vi ".vi"(0 "Array":dbl[](array[numeric]), 8 "file path (dialog if empty)":path) -> (7 "Right":cluster{"Y":dbl[], "Y":dbl[]}[](graph), 9 "Right 2":cluster{"Y":dbl[], "Y":dbl[]}[](graph), 10 "3D Graph":refnum<class "Base Datatype.lvclass">[](xcontrol), 11 "origem x":dbl, 12 "Ultimo":dbl[](array[numeric]), 13 "Roots XZ":cdb[](array[numeric]), 14 "Primeiro":dbl[](array[numeric]), 15 "origem y":dbl, 16 "Areas dos triangulos":dbl[](array[numeric]), 17 "Roots YZ":cdb[](array[numeric]), 18 "Top":cluster{"Y":dbl[], "Y":dbl[]}[](graph), 19 "Roots":cdb[](array[numeric]), 20 "chegada":dbl[](array[numeric]), 21 "Top 2":cluster{"Y":dbl[], "Y":dbl[]}[](graph), 22 "partida":dbl[](array[numeric]), 23 "Front":cluster{"Y":dbl[], "Y":dbl[]}[](graph), 24 "3D Graph 2":refnum<class "Base Datatype.lvclass">[](xcontrol), 25 "Front 2":cluster{"Y":dbl[], "Y":dbl[]}[](graph), 26 "origem z":dbl)   [LabVIEW 2019]
uses:
  <vilib>/Native 3D Graph/xcontrol/3DPC_SurfacePlot.xctl
  <vilib>/Analysis/NI_AALPro.lvlib
  <vilib>/Analysis/NI_AAL_Geometry.lvlib
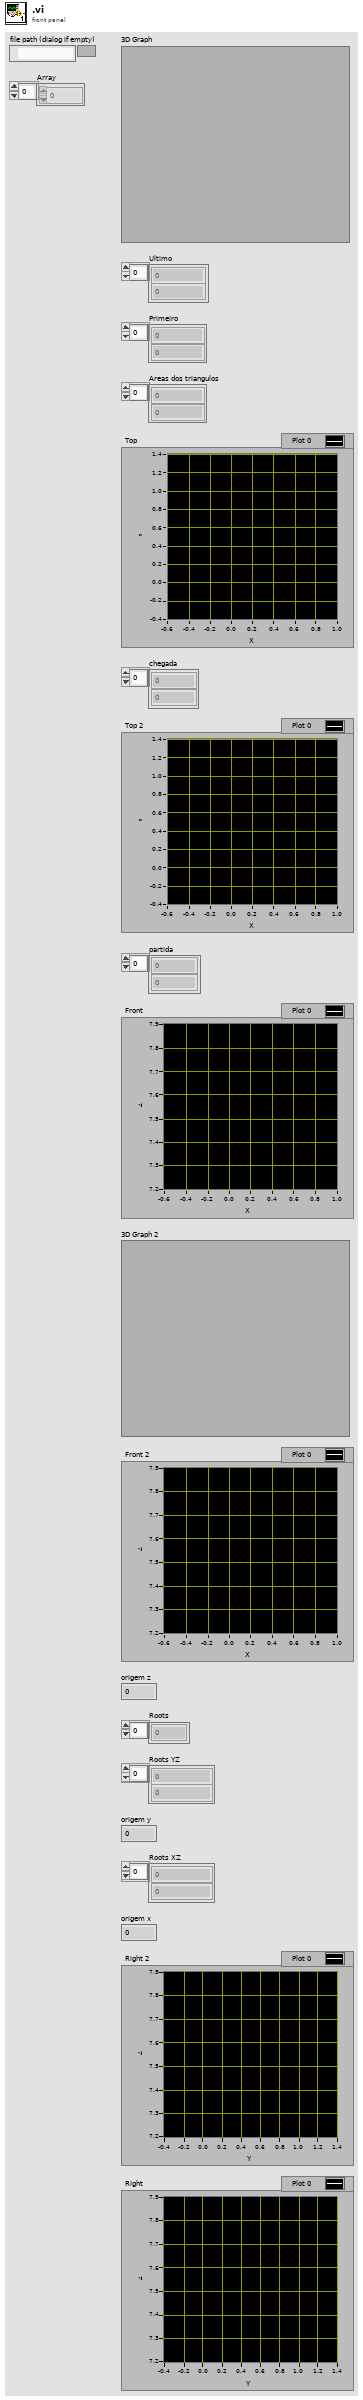
[diagram p1: front panel]
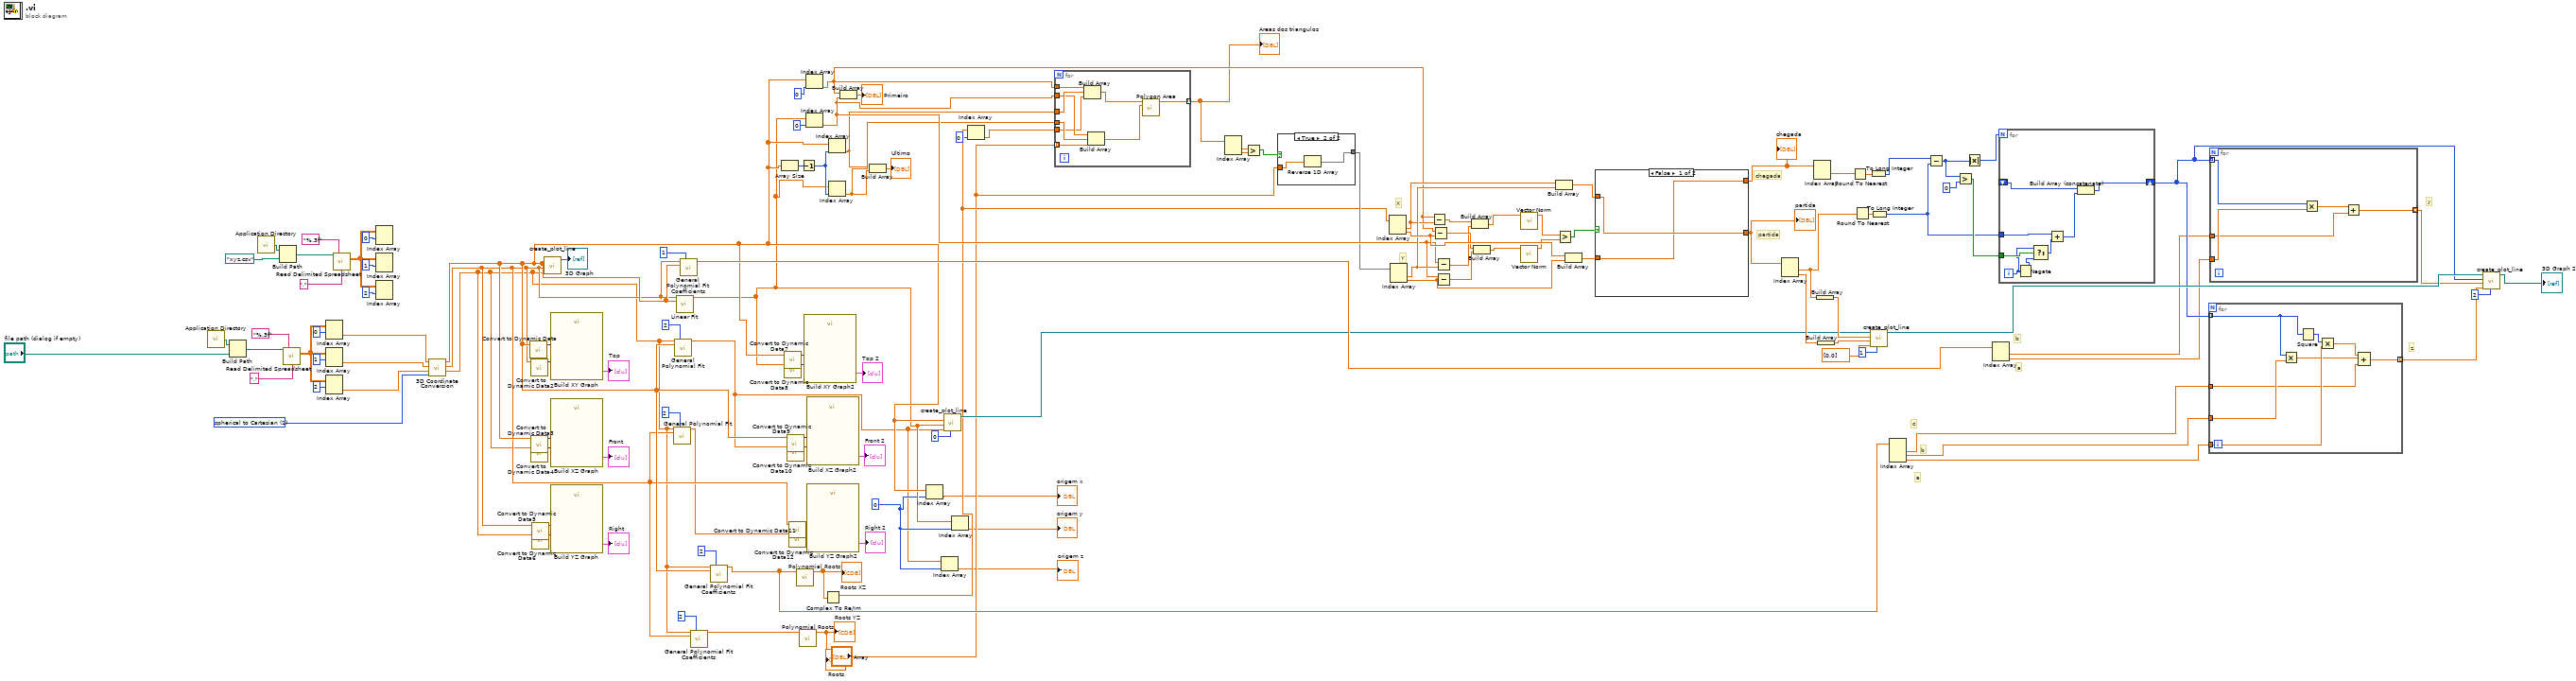
[diagram p0: block diagram]
diagram:
  w53 = 0
  w35 = u16 1 items=["Cartesian to spherical", "spherical to Cartesian", "Cartesian to cylindrical", "cylindrical to Cartesian", "spherical to cylindrical", "cylindrical to spherical"] ("conversion type")
  # "y"
  # "z"
  # "b"
  # "a"
  # "c"
  # "b"
  # "a"
  # "partida"
  # "chegada"
  # "Y"
  # "X"
  n1 = call <vilib>:"Application Directory.vi"() -> ("Application Directory"=w38:path)
  n2 = Build Path(base path=w38, name or relative path="file path (dialog if empty)") -> (appended path=w37:path)
  n3 = call <vilib>:"Application Directory.vi"() -> ("Application Directory"=w3:path)
  n4 = Build Path(base path=w3, name or relative path=path "xyz.csv" ("file path (dialog if empty)")) -> (appended path=w2:path)
  n5 = call-poly <vilib>:"Read Delimited Spreadsheet.vi"("file path (dialog if empty)"=w37, "format (%.3f)"="%.3f", "delimiter (\\t)"="," ("delimiter (\\t)")) -> ("all rows"=w44:dbl[][])  [unwired: 7 in, 5 out]
  n6 = Index Array(array=w44, index (row)=0) -> (element=w48:dbl[])  [unwired: 1 in]
  n7 = Index Array(array=w44, index (row)=1) -> (element=w47:dbl[])  [unwired: 1 in]
  n8 = Index Array(array=w44, index (row)=2) -> (element=w46:dbl[])  [unwired: 1 in]
  n9 = call-poly <vilib>:"Read Delimited Spreadsheet.vi"("file path (dialog if empty)"=w2, "format (%.3f)"="%.3f", "delimiter (\\t)"="," ("delimiter (\\t)")) -> ("all rows"=w10:dbl[][])  [unwired: 7 in, 5 out]
  n10 = Index Array(array=w10, index (row)=0) -> ()  [unwired: 1 in, 1 out]
  n11 = Index Array(array=w10, index (row)=1) -> ()  [unwired: 1 in, 1 out]
  n12 = Index Array(array=w10, index (row)=2) -> ()  [unwired: 1 in, 1 out]
  n13 = call-poly <vilib>:"3D Coordinate Conversion.vi"("conversion type"=w35, "Axis 3"=w46, "Axis 2"=w47, "Axis 1"=w48) -> ("Axis 3 Out"=w45:dbl[], "Axis 2 Out"=w112:dbl[], "Axis 1 Out"=w113:dbl[])  [unwired: 4 in, 1 out]
  n14 = call "Convert to Dynamic Data"("Array"=w113) -> ("Dynamic Data Type"=w12:dynamicdata)  [unwired: 3 in]
  n15 = call "Convert to Dynamic Data2"("Array"=w112) -> ("Dynamic Data Type"=w13:dynamicdata)  [unwired: 3 in]
  n16 = call "Convert to Dynamic Data3"("Array"=w113) -> ("Dynamic Data Type"=w16:dynamicdata)  [unwired: 3 in]
  n17 = call "Convert to Dynamic Data4"("Array"=w45) -> ("Dynamic Data Type"=w17:dynamicdata)  [unwired: 3 in]
  n18 = call "Convert to Dynamic Data5"("Array"=w112) -> ("Dynamic Data Type"=w18:dynamicdata)  [unwired: 3 in]
  n19 = call "Convert to Dynamic Data6"("Array"=w45) -> ("Dynamic Data Type"=w19:dynamicdata)  [unwired: 3 in]
  n20 = call <vilib>:"create_plot_line.vi"("z vector"=w45, "y vector"=w112, "x vector"=w113) -> ("plots out"=→"3D Graph":refnum<class "Base Datatype.lvclass">[])  [unwired: 2 in, 6 out]
  n21 = call "Build XY Graph"("Y Input"=w13, "X Input"=w12) -> ("XY Graph"=→"Top":cluster{"X":dbl[], "Y":dbl[]}[])  [unwired: 8 in, 1 out]
  n22 = call "Build XZ Graph"("Y Input"=w17, "X Input"=w16) -> ("XY Graph"=→"Front":cluster{"X":dbl[], "Y":dbl[]}[])  [unwired: 8 in, 1 out]
  n23 = call "Build YZ Graph"("Y Input"=w19, "X Input"=w18) -> ("XY Graph"=→"Right":cluster{"X":dbl[], "Y":dbl[]}[])  [unwired: 8 in, 1 out]
  n24 = call <vilib>:"General Polynomial Fit.vi"("Y"=w45, "polynomial order"=2, "X"=w112) -> ("Best Polynomial Fit"=w31:dbl[])  [unwired: 9 in, 3 out]
  n25 = call <vilib>:"General Polynomial Fit.vi"("Y"=w45, "polynomial order"=2, "X"=w113) -> ("Best Polynomial Fit"=w51:dbl[])  [unwired: 9 in, 3 out]
  n26 = call <vilib>:"Linear Fit.vi"("Y"=w112, "X"=w113) -> ("Best Linear Fit"=w56:dbl[])  [unwired: 9 in, 4 out]
  n27 = call <vilib>:"General Polynomial Fit Coefficients.vi"("Y"=w112, "polynomial order"=1, "X"=w113) -> ("Polynomial Coefficients"=w115:dbl[])  [unwired: 11 in, 1 out]
  n28 = call <vilib>:"General Polynomial Fit Coefficients.vi"("Y"=w45, "polynomial order"=2, "X"=w112) -> ("Polynomial Coefficients"=w34:dbl[])  [unwired: 11 in, 1 out]
  n29 = call <vilib>:"General Polynomial Fit Coefficients.vi"("Y"=w45, "polynomial order"=2, "X"=w113) -> ("Polynomial Coefficients"=w94:dbl[])  [unwired: 11 in, 1 out]
  n30 = Array Size(array=w113) -> (size(s)=w59:i32)
  n31 = call "Convert to Dynamic Data7"("Array"=w113) -> ("Dynamic Data Type"=w21:dynamicdata)  [unwired: 3 in]
  n32 = call "Convert to Dynamic Data8"("Array"=w56) -> ("Dynamic Data Type"=w20:dynamicdata)  [unwired: 3 in]
  n33 = call "Convert to Dynamic Data9"("Array"=w113) -> ("Dynamic Data Type"=w24:dynamicdata)  [unwired: 3 in]
  n34 = call "Convert to Dynamic Data10"("Array"=w51) -> ("Dynamic Data Type"=w23:dynamicdata)  [unwired: 3 in]
  n35 = call "Convert to Dynamic Data11"("Array"=w112) -> ("Dynamic Data Type"=w27:dynamicdata)  [unwired: 3 in]
  n36 = call "Convert to Dynamic Data12"("Array"=w31) -> ("Dynamic Data Type"=w26:dynamicdata)  [unwired: 3 in]
  n37 = call-poly <vilib>:"Polynomial Roots.vi"("P(x)"=w94) -> ("Roots"=w61:cdb[])  [unwired: 9 in, 1 out]
  "Roots XZ" <- w61
  n38 = call-poly <vilib>:"Polynomial Roots.vi"("P(x)"=w34) -> ("Roots"=→"Roots YZ" →"Roots":cdb[])  [unwired: 9 in, 1 out]
  n39 = Decrement(x=w59) -> (x-1=w60:i32)
  n40 = call "Build XY Graph2"("Y Input"=w20, "X Input"=w21) -> ("XY Graph"=→"Top 2":cluster{"X":dbl[], "Y":dbl[]}[])  [unwired: 8 in, 1 out]
  n41 = Index Array(array=w56, index=0) -> (element=w75:dbl)
  n42 = Index Array(array=w113, index=0) -> (element=w74:dbl)
  n43 = call "Build XZ Graph2"("Y Input"=w23, "X Input"=w24) -> ("XY Graph"=→"Front 2":cluster{"X":dbl[], "Y":dbl[]}[])  [unwired: 8 in, 1 out]
  n44 = call "Build YZ Graph2"("Y Input"=w26, "X Input"=w27) -> ("XY Graph"=→"Right 2":cluster{"X":dbl[], "Y":dbl[]}[])  [unwired: 8 in, 1 out]
  n45 = Complex To Re/Im(x + iy=w61) -> (x=w72:dbl[])  [unwired: 1 out]
  n46 = Index Array(array=w113, index=w60) -> (element=w63:dbl)
  n47 = Index Array(array=w56, index=w60) -> (element=w64:dbl)
  n48 = Build Array(w74, w75) -> (→"Primeiro":dbl[])
  n49 = Build Array(w63, w64) -> (→"Ultimo":dbl[])
  n50 = Index Array(array=w113, index=w53) -> (element=→"origem x":dbl)
  n51 = Index Array(array=w51, index=w53) -> (element=→"origem z":dbl)
  n52 = call <vilib>:"create_plot_line.vi"("plot ID"=0, "z vector"=w51, "y vector"=w56, "x vector"=w113) -> ("plots out"=w89:refnum<class "Base Datatype.lvclass">[])  [unwired: 1 in, 6 out]
  n53 = Index Array(array=w56, index=w53) -> (element=→"origem y":dbl)
  n54 = Index Array(array=w72, index=0) -> (element=w66:dbl)
  n55 = for {
    tunnel: "Array" -> [w130] mode=indexing
    tunnel: w74 -> [w134]
    tunnel: w75 -> [w132]
    tunnel: w63 -> [w133]
    tunnel: w64 -> [w131]
    tunnel: [w127] -> w67 mode=indexing
    tunnel: w66 -> [w126]
    n56 = Build Array(w134, w133, w126) -> (w128:dbl[])
    n57 = Build Array(w132, w131, w130) -> (w129:dbl[])
    n58 = call <vilib>:"Polygon Area.vi"("Y"=w129, "X"=w128) -> ("signed area"=w127:dbl)  [unwired: 8 in, 1 out]
  }
  "Areas dos triangulos" <- w67
  n59 = Index Array(array=w67) -> (element #1=w69:dbl, element #2=w68:dbl)  [unwired: 2 in]
  n60 = Greater?(x=w69, y=w68) -> (0:w70:bool)
  n61 = case shown="True" w70 {
    tunnel: "Array" -> [w135 w137]
    tunnel: [w135 w136] -> w73
    frame False {
    }
    frame True {
      n62 = Reverse 1D Array(array=w137) -> (reversed array=w136:dbl[])
    }
  }
  n63 = Index Array(array=w72) -> (element #1=w85:dbl, element #2=w87:dbl)  [unwired: 2 in]
  n64 = Index Array(array=w73) -> (element #1=w86:dbl, element #2=w88:dbl)  [unwired: 2 in]
  n65 = Subtract(x=w74, y=w85) -> (x-y=w76:dbl)
  n66 = Subtract(x=w74, y=w87) -> (x-y=w78:dbl)
  n67 = Subtract(x=w75, y=w86) -> (x-y=w77:dbl)
  n68 = Subtract(x=w75, y=w88) -> (x-y=w79:dbl)
  n69 = Build Array(w76, w77) -> (w83:dbl[])
  n70 = Build Array(w78, w79) -> (w84:dbl[])
  n71 = call-poly <vilib>:"Vector Norm.vi"("Input Vector"=w84) -> ("norm"=w81:dbl)  [unwired: 9 in, 1 out]
  n72 = call-poly <vilib>:"Vector Norm.vi"("Input Vector"=w83) -> ("norm"=w80:dbl)  [unwired: 9 in, 1 out]
  n73 = Build Array(w85, w86) -> (w96:dbl[])
  n74 = Greater?(x=w80, y=w81) -> (0:w82:bool)
  n75 = Build Array(w87, w88) -> (w95:dbl[])
  n76 = case shown="False" w82 {
    tunnel: [w139 w141] -> w97
    tunnel: w95 -> [w138 w141]
    tunnel: w96 -> [w139 w140]
    tunnel: [w138 w140] -> w98
    frame False {
    }
    frame True {
    }
  }
  "partida" <- w97
  "chegada" <- w98
  n77 = Index Array(array=w97) -> (element #1=w100:dbl, element #2=w91:dbl)  [unwired: 2 in]
  n78 = Index Array(array=w98) -> (element #1=w99:dbl)  [unwired: 2 in, 1 out]
  n79 = Build Array(w100) -> (w90:dbl[])
  n80 = Build Array(w91) -> (w92:dbl[])
  n81 = Round To Nearest(number=w99) -> (nearest integer value=w101:dbl)
  n82 = Round To Nearest(number=w100) -> (nearest integer value=w102:dbl)
  n83 = To Long Integer(number=w101) -> (32bit integer=w103:i32)
  n84 = call <vilib>:"create_plot_line.vi"("plot ID"=1, "z vector"=dbl[] [0.0], "y vector"=w92, "x vector"=w90, "plots in"=w89) -> ("plots out"=w121:refnum<class "Base Datatype.lvclass">[])  [unwired: 6 out]
  n85 = To Long Integer(number=w102) -> (32bit integer=w104:i32)
  n86 = Index Array(array=w94) -> (element #1=w111:dbl, element #2=w110:dbl, element #3=w109:dbl)  [unwired: 3 in]
  n87 = Subtract(x=w103, y=w104) -> (x-y=w108:i32)
  n88 = Greater?(x=w108, y=0) -> (0:w107:bool)
  n89 = Absolute Value(x=w108) -> (abs(x)=w105:i32)
  n90 = Index Array(array=w115) -> (element #1=w117:dbl, element #2=w116:dbl)  [unwired: 2 in]
  n91 = for {
    N: w105 -> [_]
    shift-right: [w146] -> w120
    shift-left: _ -> [w149]
    tunnel: w104 -> [w148]
    tunnel: w107 -> [w145]
    i -> [w143]
    n92 = Negate(x=w143) -> (-x=w144:i32)
    n93 = Select(t=w143, s=w145, f=w144) -> (s? t:f=w142:i32)
    n94 = Add(x=w148, y=w142) -> (x+y=w147:i32)
    n95 = Build Array (concatenate)(w149, w147) -> (w146:i32[])
  }
  n96 = for {
    tunnel: w109 -> [w156]
    tunnel: w110 -> [w154]
    tunnel: w111 -> [w151]
    tunnel: w120 -> [w155] mode=indexing
    tunnel: [w150] -> w118 mode=indexing
    n97 = Multiply(x=w155, y=w154) -> (x*y=w152:dbl)
    n98 = Square(x=w155) -> (x^2=w157:i32)
    n99 = Multiply(x=w157, y=w156) -> (x*y=w153:dbl)
    n100 = Compound Arithmetic op=ADD(w153, w152, w151) -> (w150:dbl)
  }
  n101 = for {
    tunnel: w120 -> [w161] mode=indexing
    tunnel: w116 -> [w162]
    tunnel: w117 -> [w160]
    tunnel: [w158] -> w119 mode=indexing
    n102 = Multiply(x=w161, y=w162) -> (x*y=w159:dbl)
    n103 = Add(x=w159, y=w160) -> (x+y=w158:dbl)
  }
  n104 = call <vilib>:"create_plot_line.vi"("plot ID"=2, "z vector"=w118, "y vector"=w119, "x vector"=w120, "plots in"=w121) -> ("plots out"=→"3D Graph 2":refnum<class "Base Datatype.lvclass">[])  [unwired: 6 out]
